vi "Decode Publish Package.vi"(7 "Type":variant, 8 "error in (no error)":errorcluster, 10 "PUBLISH":refnum<class "PUBLISH.lvclass">, 11 "MQTT_Base in":refnum<class "MQTT_Base.lvclass">) -> (0 "error out":errorcluster, 1 "Payload":variant, 2 "Topic":string, 3 "MQTT_Base out":refnum<class "MQTT_Base.lvclass">)   [LabVIEW 2013, in "MQTT Base.lvlib" / "MQTT_Base.lvclass"]
uses:
  MQTT_Base.lvclass
  <vilib>/LabVIEW Open Source Project/MQTT Control Packets/Control Packets/PUBLISH/PUBLISH.lvclass
  MQTT_Base.lvclass/MQTT_Base.ctl
  <vilib>/LabVIEW Open Source Project/MQTT Control Packets/Control Packets/ControlPacket/ControlPacket.lvclass/ControlPacket.ctl
  <vilib>/LabVIEW Open Source Project/MQTT Control Packets/Control Packets/ControlPacket/ControlPacket.lvclass
  <vilib>/LabVIEW Open Source Project/OpenSerializer/Serializer/Serializer.lvclass
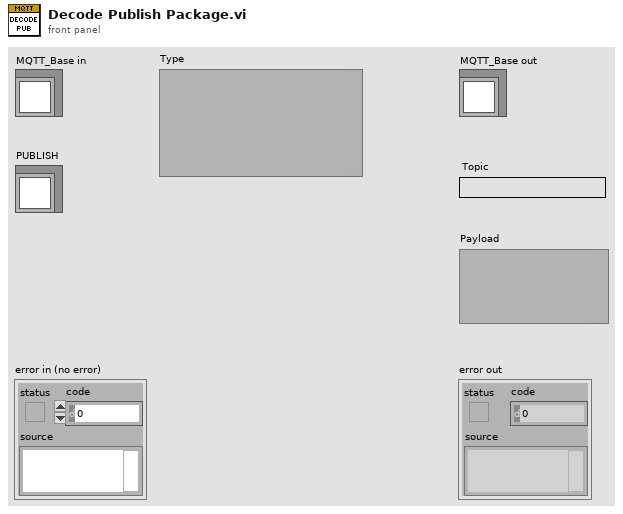
[diagram p1: front panel]
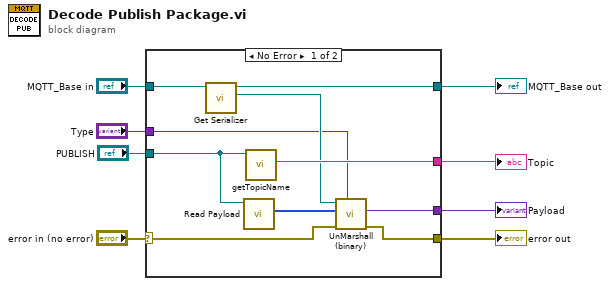
[diagram p0: block diagram]
diagram:
  n1 = case shown="No Error" "error in (no error)" {
    selector: "error in (no error)" -> [w10 w21]
    tunnel: [w9 w21] -> w7
    tunnel: [w15 w20] -> w5
    tunnel: "MQTT_Base in" -> [w16 w20]
    tunnel: "PUBLISH" -> [w17 _]
    tunnel: [w18 _] -> w3
    tunnel: [w13 w19] -> w2
    tunnel: "Type" -> [w12 w19]
    frame No Error {
      n2 = call "Get Serializer.vi"("MQTT_Base"=w16) -> ("Serializer"=w14:refnum<class "Serializer.lvclass">, "MQTT_Base out"=w15:refnum<class "MQTT_Base.lvclass">)  [unwired: 8 in, 1 out]
      n3 = call <vilib>:"Read Payload.vi"("ControlPacket in"=w17) -> ("Payload"=w11:u8[])  [unwired: 9 in, 1 out]
      n4 = call <vilib>:"getTopicName.vi"("PUBLISH in"=w17) -> ("Topic"=w18:string)  [unwired: 8 in, 2 out]
      n5 = call <vilib>:"UnMarshall (binary).vi"("Type"=w12, "error in (no error)"=w10, "Bytes"=w11, "Serializer in"=w14) -> ("error out"=w9:errorcluster, "Variant"=w13:variant)  [unwired: 5 in, 1 out]
    }
    frame Error {
    }
  }
  "error out" <- w7
  "MQTT_Base out" <- w5
  "Topic" <- w3
  "Payload" <- w2
